vi "Utility Scan Switch.vi"(0 "VISA resource name":refnum<visa-resource-name>, 7 "Scan (T: On)":bool=TRUE, 11 "error in (no error)":errorcluster) -> (4 "VISA resource name out":refnum<visa-resource-name>, 15 "error out":errorcluster)   [LabVIEW 2015, in "Chroma ATE 6310.lvlib"]
doc: "Set the scanning mode of frame to load module."
uses:
  <instrlib>/Chroma ATE 6310/Chroma ATE 6310.lvlib
panel:
  # "On\nOff"
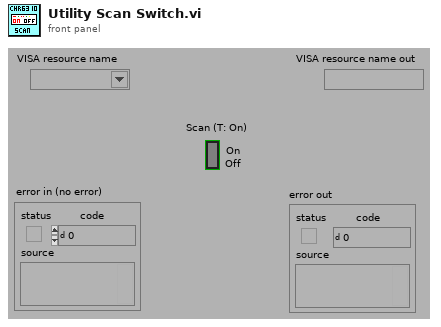
[diagram p1: front panel]
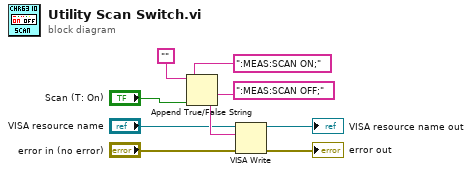
[diagram p0: block diagram]
diagram:
  n1 = Append True/False String(1:"Scan (T: On)", 2:":MEAS:SCAN OFF;", 3:":MEAS:SCAN ON;", 4:"") -> (0:w6:string)
  n2 = VISA Write(VISA resource name="VISA resource name", write buffer=w6, error in (no error)="error in (no error)") -> (VISA resource name out=→"VISA resource name out":refnum<visa-resource-name>, error out=→"error out":errorcluster)  [unwired: 1 out]
